vi "MsgMyMessage.vi"() -> (1 "MessageName":string)   [LabVIEW 2017, in "Loop3.lvlib"]
uses:
  <vilib>/addons/InsightCM/Devices/Shared/Common/DataFlow/test/SpeedBenchmark/Loop3/Loop3.lvlib
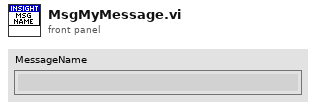
[diagram p1: front panel]
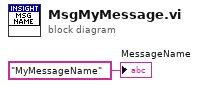
[diagram p0: block diagram]
diagram:
  "MessageName" <- "MyMessageName" ("ProcessName")
